vi "Main - Encoder.vi"() -> ()   [LabVIEW 2018]
uses:
  <vilib>/DAQmx/read.llb/DAQmx Read (Counter DBL 1Chan 1Samp).vi
  <vilib>/DAQmx/configure/timing.llb/DAQmx Timing (Implicit).vi
  <vilib>/DAQmx/write.llb/DAQmx Write (Counter 1D Frequency NChan 1Samp).vi
  typedef/Parametros control.ctl
  typedef/Selector control.ctl
panel:
  out "Tiempo de ciclo":u32
  out "Respuesta":cluster{"[0]":dbl, "[1]":dbl, "[2]":dbl}(graph)
  in  "Tipo de control":T1
  in  "Configuración":T2={"Setpoint"=0.0, "Variable de proceso"=0.0, "Frecuencia PWM"=50.0, "Ciclo de trabajo PWM"=0.5000025, "V. histeresis (grados)"=0.0, "Ganacias PID"={"proportional gain (Kc)"=1.0, "integral time (Ti, min)"=inf, "derivative time (Td, min)"=0.0}} {"Variable de proceso" min=2.5e-06 max=1.0 step=0.1; "V. histeresis (grados)" min=2.5e-06 max=0.99 step=0.01}
  in  "Setpoint":dbl(knob) scale=-170.0..170.0
  out "Variable de proceso":dbl(knob) scale=-180.0..180.0
  in  "stop":bool
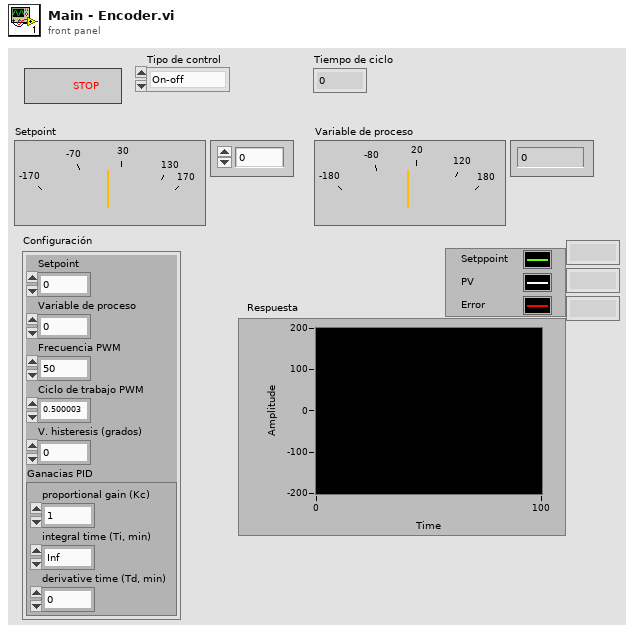
[diagram p1: front panel]
types:
  T1 = typedef "Selector control.ctl" = enum16{"On-off", "On-off hist.", "PID"}
  T2 = typedef "Parametros control.ctl" = cluster{"Setpoint":dbl, "Variable de proceso":dbl, "Frecuencia PWM":dbl, "Ciclo de trabajo PWM":dbl, "V. histeresis (grados)":dbl, "Ganacias PID":cluster{"proportional gain (Kc)":dbl, "integral time (Ti, min)":dbl, "derivative time (Td, min)":dbl}}
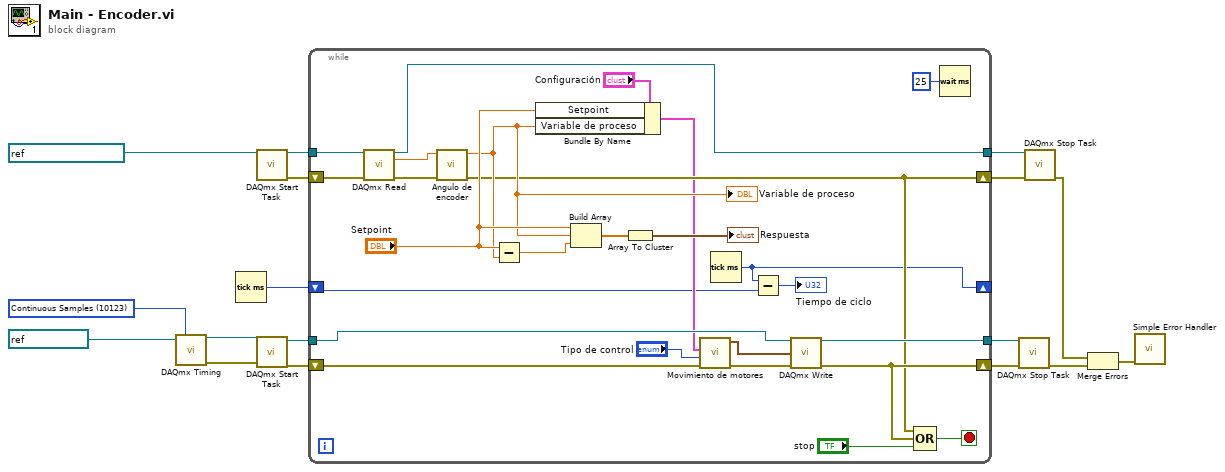
[diagram p0: block diagram]
diagram:
  w8 = 10123 items=["Finite Samples"=10178, "Continuous Samples"=10123, "Hardware Timed Single Point"=12522] ("sample mode")
  n1 = call-poly <vilib>:"DAQmx Timing.vi"("task/channels in"=refnum<k21> "CW, CCW" ("DAQmx Global Channel"), "sample mode"=w8) -> ("task out"=w10:refnum<k21>, "error out"=w9:errorcluster)  [unwired: 12 in]
  n2 = Tick Count (ms)() -> (millisecond timer value=w1:u32)
  n3 = call <vilib>:"DAQmx Start Task.vi"("task/channels in"=refnum<k21> "Posicion angular" ("DAQmx Task Name")) -> ("task out"=w17:refnum<k21>, "error out"=w16:errorcluster)  [unwired: 13 in]
  n4 = call <vilib>:"DAQmx Start Task.vi"("task/channels in"=w10, "error in"=w9) -> ("task out"=w13:refnum<k21>, "error out"=w12:errorcluster)  [unwired: 12 in]
  n5 = while {
    tunnel: w17 -> [w42]
    tunnel: [w24] -> w14
    tunnel: w13 -> [w38]
    tunnel: [w34] -> w6
    shift-right: [w35] -> w7
    shift-left: w12 -> [w39]
    shift-right: [w22] -> w15
    shift-left: w16 -> [w40]
    shift-right: [w19] -> _
    shift-left: w1 -> [w20]
    stop <- w36 stop-if-true
    n6 = call-poly <vilib>:"DAQmx Read.vi"("task/channels in"=w42, "error in"=w40) -> ("task out"=w24:refnum<k21>, "data"=w26:dbl, "error out"=w23:errorcluster)  [unwired: 11 in]
    n7 = call "Angulo de encoder.vi"("error in (no error)"=w23, "Input angle"=w26) -> ("error out"=w22:errorcluster, "Output angle"=w25:dbl)  [unwired: 8 in]
    "Variable de proceso" <- w25
    n8 = Subtract(x="Setpoint", y=w25) -> (x-y=w30:dbl)
    n9 = Bundle By Name(cluster="Configuración", "Setpoint"="Setpoint", "Variable de proceso"=w25) -> (w21:T2)
    n10 = Build Array("Setpoint", w25, w30) -> (w32:dbl[])
    n11 = Array To Cluster(array=w32) -> (cluster=→"Respuesta":cluster{"[0]":dbl, "[1]":dbl, "[2]":dbl})
    n12 = call "Movimiento de motores.vi"("Tipo de control"="Tipo de control", "Parametros de control"=w21) -> ("Salida a motores"=w37:cluster{"duty cycle":dbl, "frequency":dbl}[])  [unwired: 8 in, 1 out]
    n13 = Tick Count (ms)() -> (millisecond timer value=w19:u32)
    n14 = Subtract(x=w19, y=w20) -> (x-y=→"Tiempo de ciclo":u32)
    n15 = call-poly <vilib>:"DAQmx Write.vi"("task/channels in"=w38, "data"=w37, "error in"=w39) -> ("task out"=w34:refnum<k21>, "error out"=w35:errorcluster)  [unwired: 10 in, 1 out]
    n16 = Compound Arithmetic op=OR(w22, w35, "stop") -> (w36:bool)
    n17 = Wait (ms)(milliseconds to wait=u32 25) -> ()  [unwired: 1 out]
  }
  n18 = call <vilib>:"DAQmx Stop Task.vi"("task/channels in"=w6, "error in"=w7) -> ("error out"=w5:errorcluster)  [unwired: 12 in, 1 out]
  n19 = call <vilib>:"DAQmx Stop Task.vi"("task/channels in"=w14, "error in"=w15) -> ("error out"=w4:errorcluster)  [unwired: 12 in, 1 out]
  n20 = Merge Errors(w4, w5) -> (w3:errorcluster)
  n21 = call <vilib>:"Simple Error Handler.vi"("error in (no error)"=w3) -> ()  [unwired: 4 in, 5 out]
